vi "Do Charact.vi"(0 "Vector Path in":refnum<class "Vector 18GHz Path.lvclass">, 5 "Standard Type":T1, 11 "error in":errorcluster) -> (4 "Vector Path out":refnum<class "Vector 18GHz Path.lvclass">, 6 "Aborted":bool, 15 "error out":errorcluster)   [LabVIEW 2023, in "RFFixtureCharact.RFPM.lvlib" / "Vector 18GHz Path.lvclass"]
uses:
  Vector 18GHz Path.lvclass
  Instruments/Cal Standard/Type Definitions/Standard Type.ctl
  Vector 18GHz Path.lvclass/Vector 18GHz Path.ctl
  Instruments/RFFixtureCharact.Instruments.lvlib
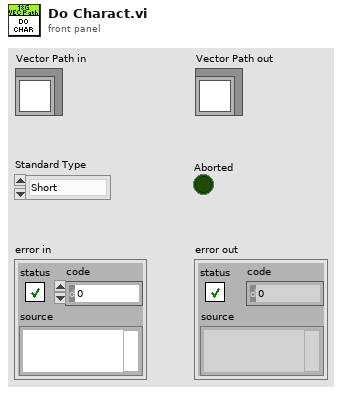
[diagram p1: front panel]
types:
  T1 = typedef "RFFixtureCharact.Instruments.lvlib/Standard Type.ctl" = enum16{"Short", "Open", "Load", "PowerMeter", "None"}
  T2 = typedef "RFFixtureCharact.Instruments.lvlib/One-Port Charact Data.ctl" = cluster{"Standard Type":T1, "Frequencies":dbl[], "S11":cdb[]}
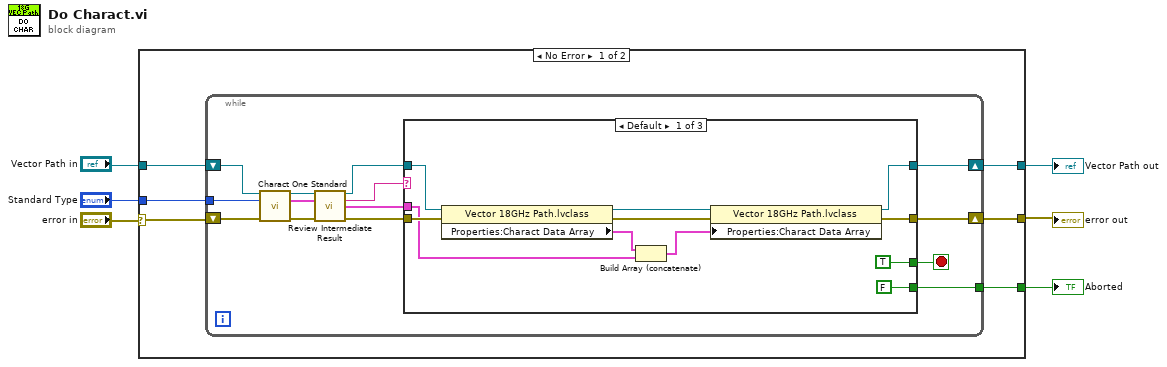
[diagram p0: block diagram]
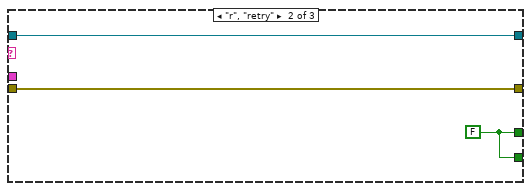
[diagram p2: hidden frame]
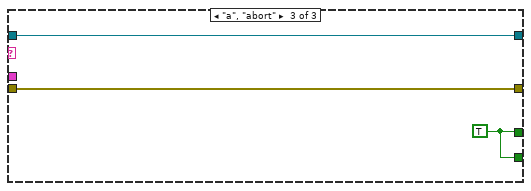
[diagram p3: hidden frame]
diagram:
  n1 = case shown="No Error" "error in" {
    selector: "error in" -> [w9 w45]
    tunnel: "Vector Path in" -> [w8 w44]
    tunnel: [w11 w45] -> w2
    tunnel: [w12 w44] -> w1
    tunnel: "Standard Type" -> [w7 _]
    tunnel: [w10 _] -> w3
    frame No Error {
      n2 = while {
        shift-right: [w20] -> w11
        shift-left: w9 -> [w26]
        shift-right: [w22] -> w12
        shift-left: w8 -> [w25]
        tunnel: [w23] -> w10
        tunnel: w7 -> [w19]
        stop <- w24 stop-if-true
        n3 = call-dynamic "Charact One Standard.vi"("Vector Path in"=w25, "Standard Type"=w19, "error in"=w26) -> ("Vector Path out"=w17:refnum<class "Vector 18GHz Path.lvclass">, "One-Port Charact Data"=w13:T2, "error out"=w18:errorcluster)  [unwired: 10 in]
        n4 = call-dynamic "Review Intermediate Result.vi"("Vector 18GHz Path in"=w17, "One-Port Charact Data In"=w13, "error in (no error)"=w18) -> ("Vector 18GHz Path out"=w16:refnum<class "Vector 18GHz Path.lvclass">, "Response"=w15:string, "One-Port Charact Data Out"=w14:T2, "error out"=w21:errorcluster)  [unwired: 9 in]
        n5 = case shown="Default" w15 {
          tunnel: [TRUE w38 w41] -> w24
          tunnel: [FALSE w38 w41] -> w23
          tunnel: [w31 w40 w43] -> w22
          tunnel: w16 -> [w36 w40 w43]
          tunnel: w21 -> [w35 w39 w42]
          tunnel: [w30 w39 w42] -> w20
          tunnel: w14 -> [w33 _ _]
          frame Default {
            n6 = property class="Vector 18GHz Path.lvclass"(reference=w36, error in=w35) -> (reference out=w32:refnum<class "Vector 18GHz Path.lvclass">, error out=w29:errorcluster, "Properties:Charact Data Array"=w34:T2[])
            n7 = Build Array (concatenate)(w34, w33) -> (w28:T2[])
            n8 = property class="Vector 18GHz Path.lvclass"(reference=w32, error in=w29, "Properties:Charact Data Array"=w28) -> (reference out=w31:refnum<class "Vector 18GHz Path.lvclass">, error out=w30:errorcluster)
          }
          frame "r", "retry" {
            w38 = FALSE
          }
          frame "a", "abort" {
            w41 = TRUE
          }
        }
      }
    }
    frame Error {
    }
  }
  "error out" <- w2
  "Vector Path out" <- w1
  "Aborted" <- w3
